vi "NodeUI.vi"() -> ()   [LabVIEW 2023, in "CEF.lvlib" / "CEF_Node.lvclass"]
doc: "UI that will be called when the node is selected.Copyright 2017 National Instruments Corporation\n\nLicensed under the Apache License, Version 2.0 (the \"License\"); you may not use this file except in compliance with the License. You may obtain a copy of the License at http://www.apache.org/licenses/LICENSE-2.0\nUnless required by applicable law or agreed to in writing, software distributed under the License is distributed on an \"AS IS\" BASIS, WITHOUT WARRANTIES OR CONDITIONS OF ANY KIND, either express or implied. See the License for the specific language governing permissions and limitations under the License."
uses:
  CEF_Node.lvclass
  NodeRef.ctl
  mainQref.ctl
  Message.ctl
  UserEventRef.ctl
  Controls/EventCluster.ctl
  RefreshUIEvent.ctl
  CacheState.ctl
  StopEvent.ctl
  NodeChangeEvent.ctl
  CEF.lvlib
panel:
  in  "node change":T1
  in  "stop event":T2
  in  "cache state":T3
  in  "refresh UI":T4
  out "Loop Counter":i32
  in  "user event":T5
  in  "main queue":T6
  in  "String":string
  in  "node ref":T7
  # "Default node UI\nNo UI has been created for this type of node."
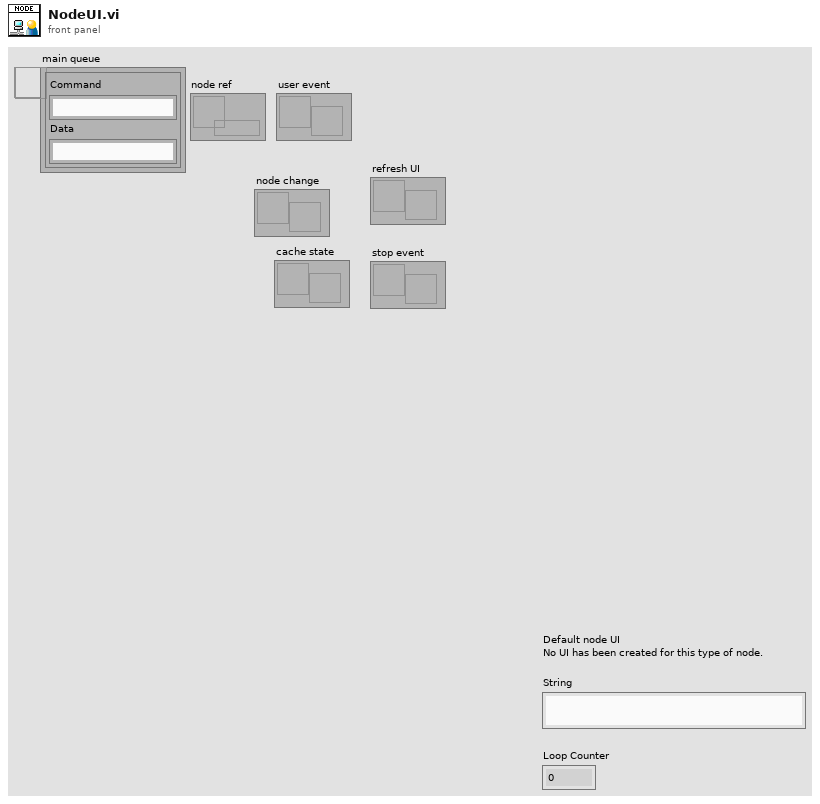
[diagram p1: front panel]
types:
  T1 = typedef "CEF.lvlib/CEF_Node.lvclass/NodeChangeEvent.ctl" = refnum<user-event>
  T2 = typedef "CEF.lvlib/CEF_Node.lvclass/StopEvent.ctl" = refnum<user-event>
  T3 = typedef "CEF.lvlib/CEF_Node.lvclass/CacheState.ctl" = refnum<user-event>
  T4 = typedef "CEF.lvlib/CEF_Node.lvclass/RefreshUIEvent.ctl" = refnum<user-event>
  T5 = typedef "CEF.lvlib/CEF_Node.lvclass/UserEventRef.ctl" = refnum<user-event>
  T6 = typedef "CEF.lvlib/CEF_Node.lvclass/mainQref.ctl" = refnum<queue>
  T7 = typedef "CEF.lvlib/CEF_Node.lvclass/NodeRef.ctl" = refnum<data-value>
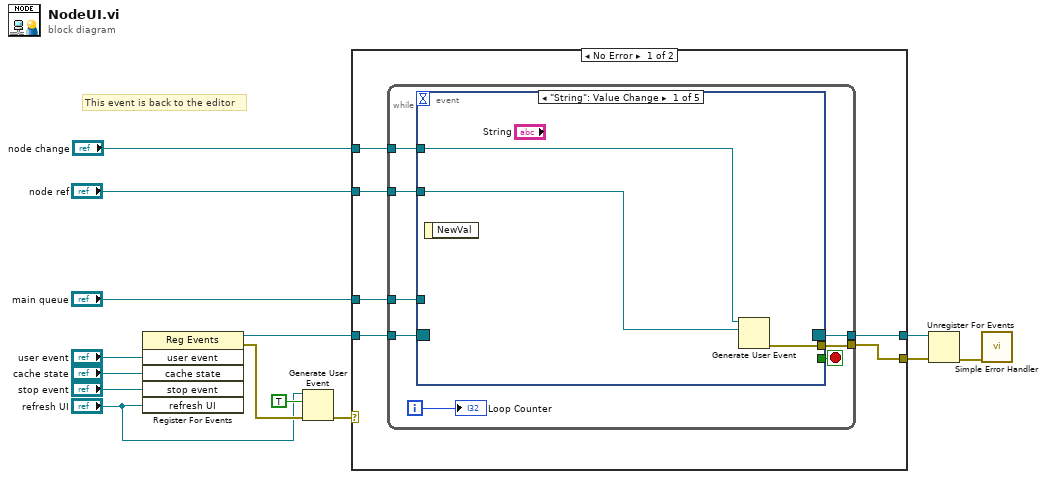
[diagram p0: block diagram]
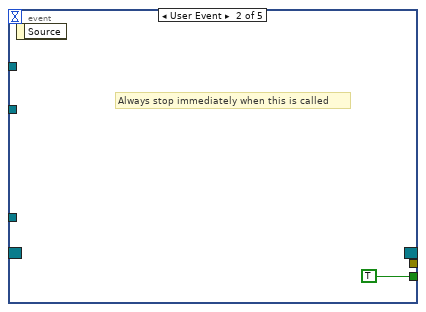
[diagram p2: hidden frame]
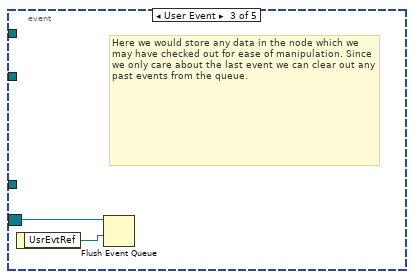
[diagram p3: hidden frame]
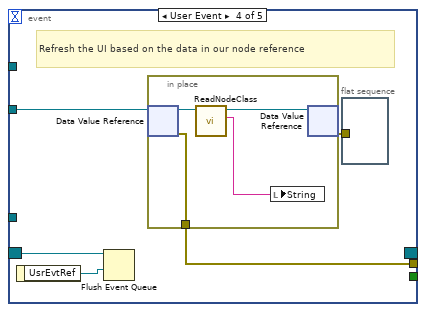
[diagram p4: hidden frame]
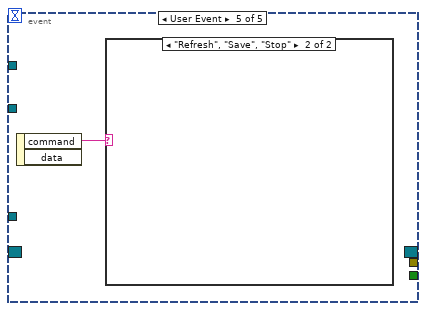
[diagram p5: hidden frame]
diagram:
  # "This event is back to the editor"
  n1 = register-events("user event", "cache state", "stop event", "refresh UI") -> (reference out=w12:refnum<event-registration>, error out=w9:errorcluster)  [unwired: 2 in]
  n2 = Generate User Event(user event="refresh UI", event data cluster=TRUE ("event data"), error in=w9) -> (error out=w7:errorcluster)  [unwired: 1 in, 1 out]
  n3 = case shown="No Error" w7 {
    selector: w7 -> [_ w46]
    tunnel: "node ref" -> [w20 _]
    tunnel: "main queue" -> [w19 _]
    tunnel: w12 -> [w18 w45]
    tunnel: [w17 w45] -> w11
    tunnel: [w16 w46] -> w10
    tunnel: "node change" -> [w15 _]
    frame No Error {
      n4 = while {
        tunnel: w20 -> [w28]
        tunnel: w19 -> [w27]
        tunnel: w18 -> [w26]
        tunnel: [w25] -> w17
        tunnel: [w24] -> w16
        tunnel: w15 -> [w21]
        i -> [w23]
        stop <- w22 stop-if-true
        n5 = event shown="[0] \"String\": Value Change" {
          selector: w26 -> [_ _ w34 w39 _]
          dyn-events: [_ _ _ _ _] -> w25
          timeout: _ -> [_ _ _ _ _]
          tunnel: w28 -> [w29 _ _ w35 _]
          tunnel: w27 -> [_ _ _ _ _]
          tunnel: [w31 _ _ w36 _] -> w24
          tunnel: [_ TRUE _ _ _] -> w22
          tunnel: w21 -> [w30 _ _ _ _]
          event "String": Value Change {
            n6 = event-data() -> ()  [unwired: 1 in, 1 out]
            n7 = Generate User Event(user event=w30, event data cluster=w29) -> (error out=w31:errorcluster)  [unwired: 2 in, 1 out]
          }
          event User Event {
            # "Always stop immediately when this is called"
            n8 = event-data() -> ()  [unwired: 1 in, 1 out]
          }
          event User Event {
            # "Here we would store any data in the node which we may have checked out for ease of manipulation. Since we only care about the last event we can clear out any past events from the queue."
            n9 = event-data() -> ("UsrEvtRef"=w33:refnum<user-event>)  [unwired: 1 in]
            n10 = Flush Event Queue(0:w34, 2:w33) -> ()  [unwired: 4 in, 3 out]
          }
          event User Event {
            # "Refresh the UI based on the data in our node reference"
            n11 = event-data() -> ("UsrEvtRef"=w38:refnum<user-event>)  [unwired: 1 in]
            n12 = Flush Event Queue(0:w39, 2:w38) -> ()  [unwired: 4 in, 3 out]
            n13 = in-place {
              in-place-border: [w40] -> w36
              n14 = in-place-dvr #1(w35) -> (w43:refnum<class "CEF_Node.lvclass">, w40:errorcluster)
              n15 = call "ReadNodeClass.vi"("node in"=w43) -> ("nodeClass"=w41:string, "node out"=w42:refnum<class "CEF_Node.lvclass">)  [unwired: 8 in, 1 out]
              n16 = local write "String"(w41) -> ()
              n17 = in-place-dvr #1(w42) -> (w37:errorcluster)  [unwired: 1 out]
            }
            n18 = flat-sequence {
              tunnel: w37 -> [_]
              frame #0 {
              }
            }
          }
          event User Event {
            n19 = event-data() -> ("command"=w44:string)  [unwired: 1 in, 1 out]
            n20 = case shown="\"Refresh\", \"Save\", \"Stop\"" w44 {
              frame Default {
                # "Use this case for any user-specified events\n\nFor legacy compatibility the framework will still trigger this event with the message \"Stop\", \"Refresh\", and \"Save\". However, since we have registered for the new specific events we can ignore framework events here."
              }
              frame "Refresh", "Save", "Stop" {
              }
            }
          }
        }
        "Loop Counter" <- w23
      }
    }
    frame Error {
    }
  }
  n21 = Unregister For Events(event registration refnum=w11, error in=w10) -> (error out=w6:errorcluster)
  n22 = call <vilib>:"Simple Error Handler.vi"("error in (no error)"=w6) -> ()  [unwired: 4 in, 5 out]
